vi "4Pi Capture Scan Counter.vi"(8 "Scan Tracker":T1) -> (0 "Scan Tracker Out":T1, 1 "Move stage?":bool, 2 "F_MVR/T_MOV":bool, 3 "Exit?":bool)   [LabVIEW 2016]
uses:
  4Pi Capture Manager Controls/4Pi Capture Scan Tracker.ctl
  4Pi Capture Manager Controls/4Pi Capture Switch Laser.ctl
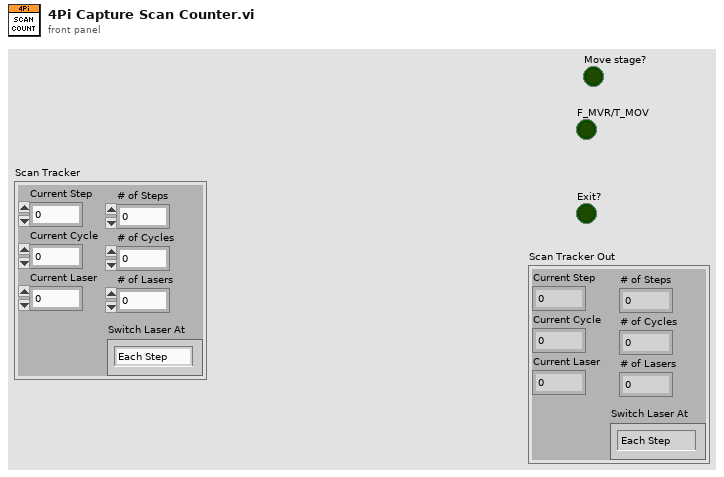
[diagram p1: front panel]
types:
  T1 = typedef "4Pi Capture Scan Tracker.ctl" = cluster{"Current Step":u16, "Current Cycle":u16, "Current Laser":u16, "# of Lasers":u16, "# of Cycles":u16, "# of Steps":u16, "Switch Laser At":T2}
  T2 = typedef "4Pi Capture Switch Laser.ctl" = enum16{"Each Step", "Each Cycle", "All Cycles"}
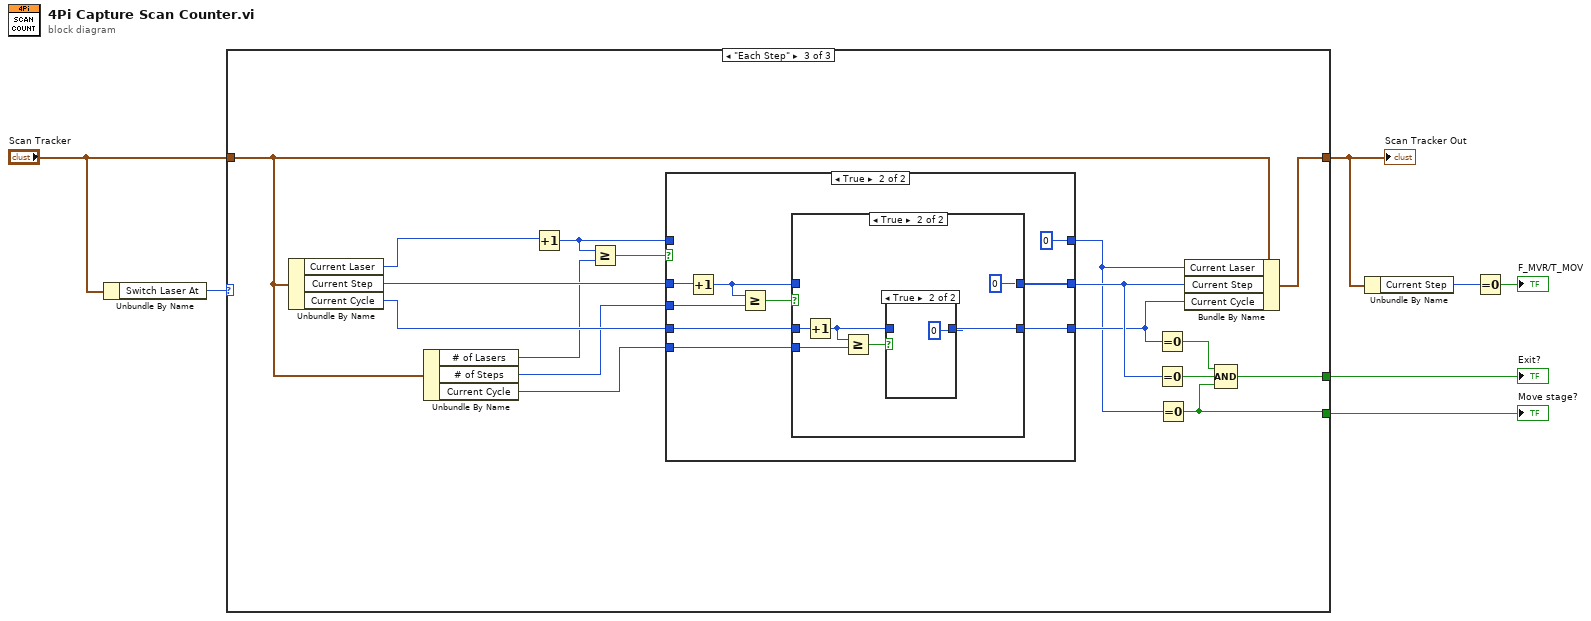
[diagram p0: block diagram]
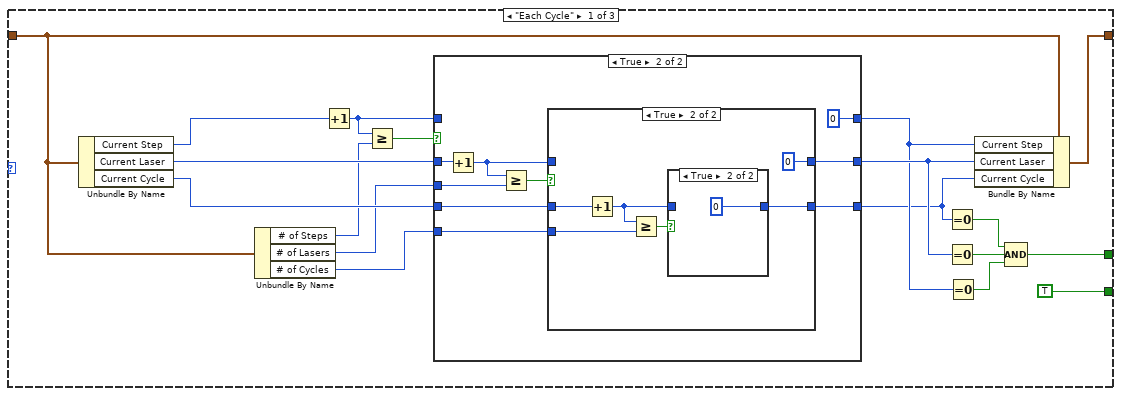
[diagram p2: hidden frame]
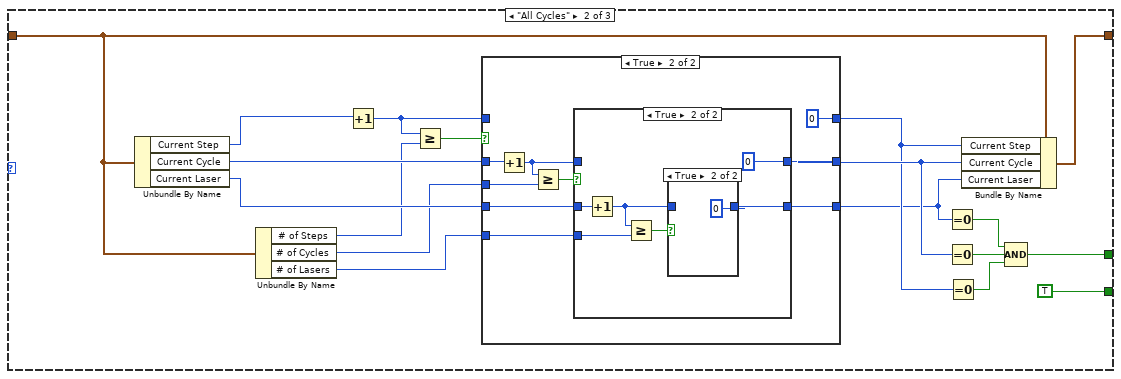
[diagram p6: hidden frame]
diagram:
  n1 = Unbundle By Name("Scan Tracker") -> ("Switch Laser At"=w7:T2)
  n2 = case shown="\"Each Step\"" w7 {
    tunnel: "Scan Tracker" -> [w9 w48 w88]
    tunnel: [w14 w53 w95] -> w3
    tunnel: [w13 w52 w94] -> w6
    tunnel: [TRUE TRUE w89] -> w2
    frame "Each Cycle" {
      n3 = Unbundle By Name(w9) -> ("Current Step"=w8:u16, "Current Laser"=w25:u16, "Current Cycle"=w24:u16)
      n4 = Unbundle By Name(w9) -> ("# of Steps"=w11:u16, "# of Lasers"=w22:u16, "# of Cycles"=w21:u16)
      n5 = Increment(x=w8) -> (x+1=w12:u16)
      n6 = Greater Or Equal?(x=w12, y=w11) -> (x >= y?=w23:bool)
      n7 = case shown="True" w23 {
        tunnel: [w28 u16 0] -> w19
        tunnel: w12 -> [w28 _]
        tunnel: w25 -> [w27 w37]
        tunnel: w24 -> [w26 w32]
        tunnel: w22 -> [_ w29]
        tunnel: [w27 w34] -> w20
        tunnel: w21 -> [_ w33]
        tunnel: [w26 w31] -> w18
        frame False {
        }
        frame True {
          n8 = Increment(x=w37) -> (x+1=w30:u16)
          n9 = Greater Or Equal?(x=w30, y=w29) -> (x >= y?=w36:bool)
          n10 = case shown="True" w36 {
            tunnel: [w39 u16 0] -> w34
            tunnel: w30 -> [w39 _]
            tunnel: w33 -> [_ w40]
            tunnel: w32 -> [w38 w44]
            tunnel: [w38 w43] -> w31
            frame False {
            }
            frame True {
              n11 = Increment(x=w44) -> (x+1=w41:u16)
              n12 = Greater Or Equal?(x=w41, y=w40) -> (x >= y?=w45:bool)
              n13 = case shown="True" w45 {
                tunnel: [w46 u16 0] -> w43
                tunnel: w41 -> [w46 _]
                frame False {
                }
                frame True {
                }
              }
            }
          }
        }
      }
      n14 = Equal To 0?(x=w18) -> (x = 0?=w17:bool)
      n15 = Equal To 0?(x=w20) -> (x = 0?=w16:bool)
      n16 = Equal To 0?(x=w19) -> (x = 0?=w15:bool)
      n17 = Bundle By Name(cluster=w9, "Current Step"=w19, "Current Laser"=w20, "Current Cycle"=w18) -> (w13:T1)
      n18 = Compound Arithmetic op=AND(w17, w16, w15) -> (w14:bool)
    }
    frame "All Cycles" {
      n19 = Unbundle By Name(w48) -> ("Current Step"=w65:u16, "Current Cycle"=w64:u16, "Current Laser"=w63:u16)
      n20 = Unbundle By Name(w48) -> ("# of Steps"=w50:u16, "# of Cycles"=w61:u16, "# of Lasers"=w60:u16)
      n21 = Increment(x=w65) -> (x+1=w51:u16)
      n22 = Greater Or Equal?(x=w51, y=w50) -> (x >= y?=w62:bool)
      n23 = case shown="True" w62 {
        tunnel: [w68 u16 0] -> w58
        tunnel: w51 -> [w68 _]
        tunnel: w64 -> [w67 w77]
        tunnel: w63 -> [w66 w72]
        tunnel: w61 -> [_ w70]
        tunnel: [w67 w74] -> w59
        tunnel: w60 -> [_ w73]
        tunnel: [w66 w71] -> w57
        frame False {
        }
        frame True {
          n24 = Increment(x=w77) -> (x+1=w69:u16)
          n25 = Greater Or Equal?(x=w69, y=w70) -> (x >= y?=w76:bool)
          n26 = case shown="True" w76 {
            tunnel: [w79 u16 0] -> w74
            tunnel: w69 -> [w79 _]
            tunnel: w73 -> [_ w81]
            tunnel: w72 -> [w78 w84]
            tunnel: [w78 w83] -> w71
            frame False {
            }
            frame True {
              n27 = Increment(x=w84) -> (x+1=w80:u16)
              n28 = Greater Or Equal?(x=w80, y=w81) -> (x >= y?=w85:bool)
              n29 = case shown="True" w85 {
                tunnel: [w86 u16 0] -> w83
                tunnel: w80 -> [w86 _]
                frame False {
                }
                frame True {
                }
              }
            }
          }
        }
      }
      n30 = Equal To 0?(x=w57) -> (x = 0?=w56:bool)
      n31 = Equal To 0?(x=w59) -> (x = 0?=w55:bool)
      n32 = Equal To 0?(x=w58) -> (x = 0?=w54:bool)
      n33 = Bundle By Name(cluster=w48, "Current Step"=w58, "Current Cycle"=w59, "Current Laser"=w57) -> (w52:T1)
      n34 = Compound Arithmetic op=AND(w56, w55, w54) -> (w53:bool)
    }
    frame "Each Step" {
      n35 = Unbundle By Name(w88) -> ("Current Laser"=w104:u16, "Current Step"=w103:u16, "Current Cycle"=w102:u16)
      n36 = Unbundle By Name(w88) -> ("# of Lasers"=w92:u16, "# of Steps"=w91:u16, "Current Cycle"=w100:u16)
      n37 = Increment(x=w104) -> (x+1=w93:u16)
      n38 = Greater Or Equal?(x=w93, y=w92) -> (x >= y?=w101:bool)
      n39 = case shown="True" w101 {
        tunnel: [w107 u16 0] -> w90
        tunnel: w93 -> [w107 _]
        tunnel: w103 -> [w106 w116]
        tunnel: w102 -> [w105 w111]
        tunnel: w91 -> [_ w108]
        tunnel: [w106 w113] -> w99
        tunnel: w100 -> [_ w112]
        tunnel: [w105 w110] -> w98
        frame False {
        }
        frame True {
          n40 = Increment(x=w116) -> (x+1=w109:u16)
          n41 = Greater Or Equal?(x=w109, y=w108) -> (x >= y?=w115:bool)
          n42 = case shown="True" w115 {
            tunnel: [w118 u16 0] -> w113
            tunnel: w109 -> [w118 _]
            tunnel: w112 -> [_ w119]
            tunnel: w111 -> [w117 w123]
            tunnel: [w117 w122] -> w110
            frame False {
            }
            frame True {
              n43 = Increment(x=w123) -> (x+1=w120:u16)
              n44 = Greater Or Equal?(x=w120, y=w119) -> (x >= y?=w124:bool)
              n45 = case shown="True" w124 {
                tunnel: [w125 u16 0] -> w122
                tunnel: w120 -> [w125 _]
                frame False {
                }
                frame True {
                }
              }
            }
          }
        }
      }
      n46 = Equal To 0?(x=w98) -> (x = 0?=w97:bool)
      n47 = Equal To 0?(x=w99) -> (x = 0?=w96:bool)
      n48 = Equal To 0?(x=w90) -> (x = 0?=w89:bool)
      n49 = Bundle By Name(cluster=w88, "Current Laser"=w90, "Current Step"=w99, "Current Cycle"=w98) -> (w94:T1)
      n50 = Compound Arithmetic op=AND(w97, w96, w89) -> (w95:bool)
    }
  }
  "Exit?" <- w3
  "Move stage?" <- w2
  "Scan Tracker Out" <- w6
  n51 = Unbundle By Name(w6) -> ("Current Step"=w5:u16)
  n52 = Equal To 0?(x=w5) -> (x = 0?=→"F_MVR/T_MOV":bool)
